vi "TestCloneAPI.vi"() -> ()   [LabVIEW 2018, in "MyPluggableModule.lvlib"]
uses:
  MyPluggableModule.lvlib
  TestInfo.ctl
  <userlib>/NIST/ModuleAdminLib/CloneRegistration/CloneRegistration.lvclass
  <userlib>/NIST/ModuleAdminLib/ModuleAdmin/ModuleAdmin.lvclass/ModuleAdmin.ctl
  <userlib>/NIST/ModuleAdminLib/ModuleAdmin/ModuleAdmin.lvclass
  PluginsShared/clDidInit.ctl
  PluginsShared/clStopArgument.ctl
  <userlib>/NIST/ModuleAdminLib/ModuleAdmin/Accessors/Read CloneRegRef.vi
  <userlib>/NIST/ModuleAdminLib/ModuleAdmin/Accessors/Write CloneRegRef.vi
  PluginsShared/PluginsShared.lvlib
panel:
  in  "btnClear":bool
  in  "btnPref":bool
  in  "Show Panel":bool=TRUE
  in  "Plugin Type":u16(ring) items=["Base Plugin"]
  in  "btnLoadPlugin":bool
  out "File Path Control":path
  in  "btnRequestINIPath":bool
  in  "btnRemove":bool
  out "Status Log":string
  out "Active Modules (Array)":string[](array[string])
  in  "btnAdd":bool
  in  "btnStop":bool
  in  "Select Module":i32(ring)=-1 caption="Select Module to send Request" items=["All"=-1]
  # "Use TestCloneAPI to test the CloneableModule's Application Programming Interface as you develop it.  For each Request and Broadcast event you add to the Clone's Main program, you should add a means of testing it."
  # "Hidden"
  # "Visible"
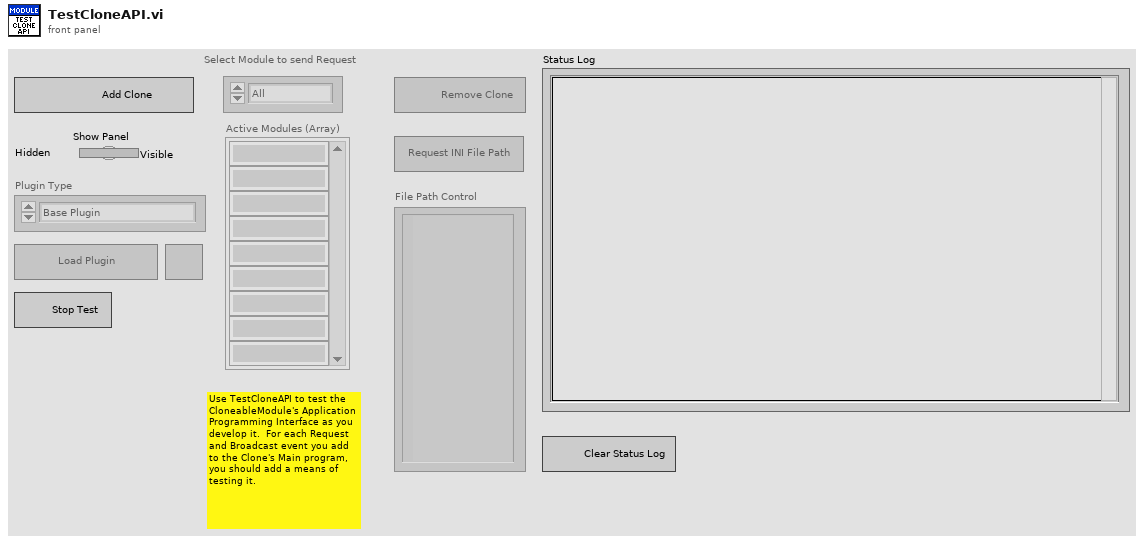
[diagram p1: front panel]
types:
  T1 = typedef "MyPluggableModule.lvlib/TestInfo.ctl" = cluster{"PluginIniFilePaths":path[]}
  T2 = cluster{"Status Log":refnum<vi>, "btnAdd":refnum<vi>, "btnStop":refnum<vi>, "Show Panel":refnum<vi>, "btnClear":refnum<vi>}
  T3 = typedef "PluginsShared.lvlib/clBroadcastEvents.ctl" = cluster{"DidInit":refnum<user-event>, "StatusUpdate":refnum<user-event>, "ErrorReport":refnum<user-event>, "DidStop":refnum<user-event>, "PathToINI":refnum<user-event>, "ReloadINIFiles":refnum<user-event>}
  T4 = enum8{"Enabled", "Disabled", "Disabled and Grayed Out"}
  T5 = typedef "PluginsShared.lvlib/clDidInit.ctl" = cluster{"Init?":bool, "ModuleAdmin":refnum<class "ModuleAdmin.lvclass">}
  T6 = typedef "PluginsShared.lvlib/clStopArgument.ctl" = cluster{"Exit via Stop Module Req?":bool, "Wait for Module to stop?":bool, "ModuleAdmin":refnum<class "ModuleAdmin.lvclass">}
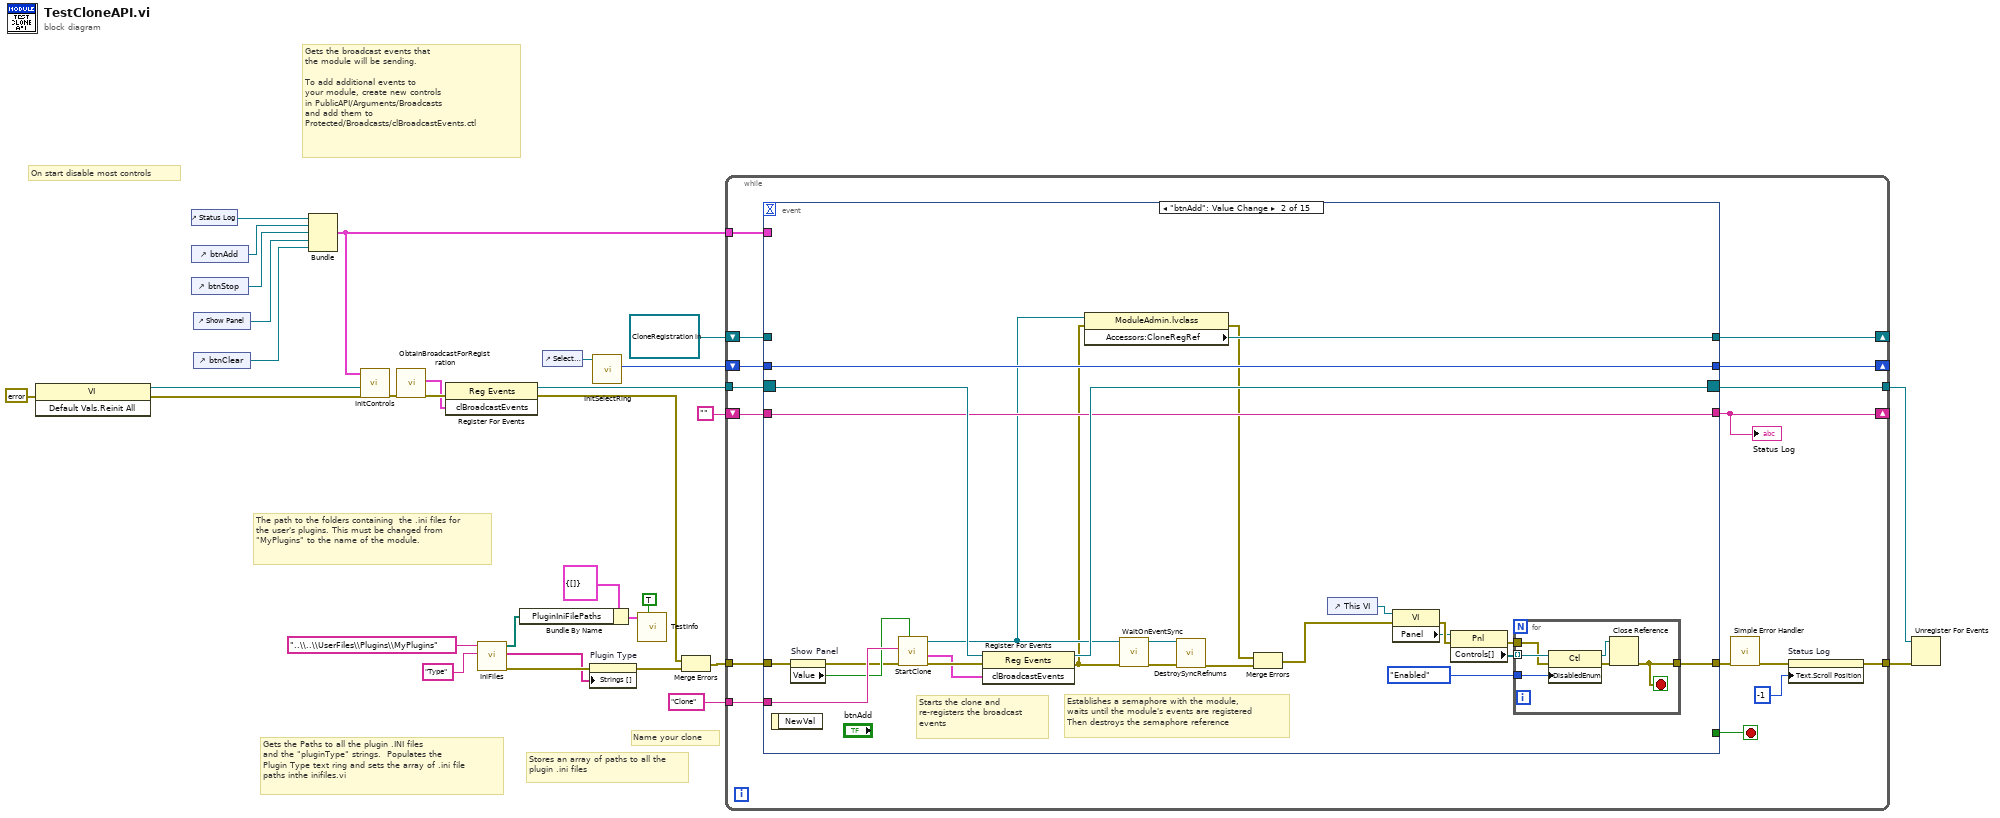
[diagram p0: block diagram]
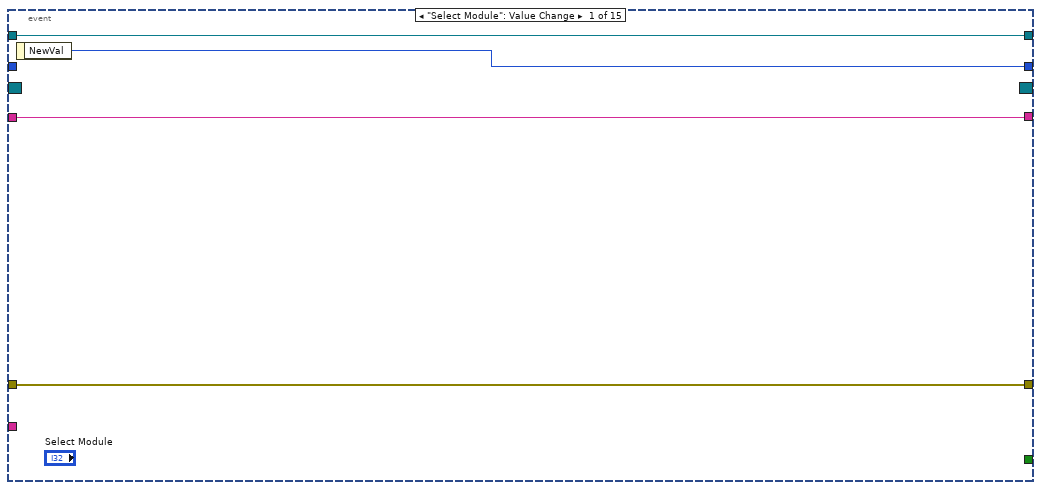
[diagram p2: hidden frame]
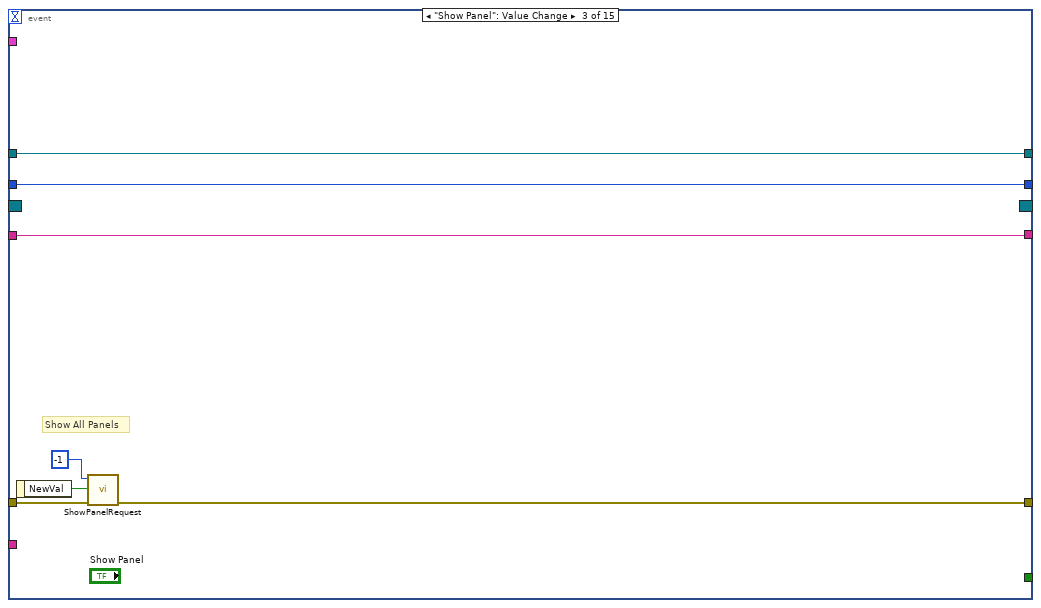
[diagram p3: hidden frame]
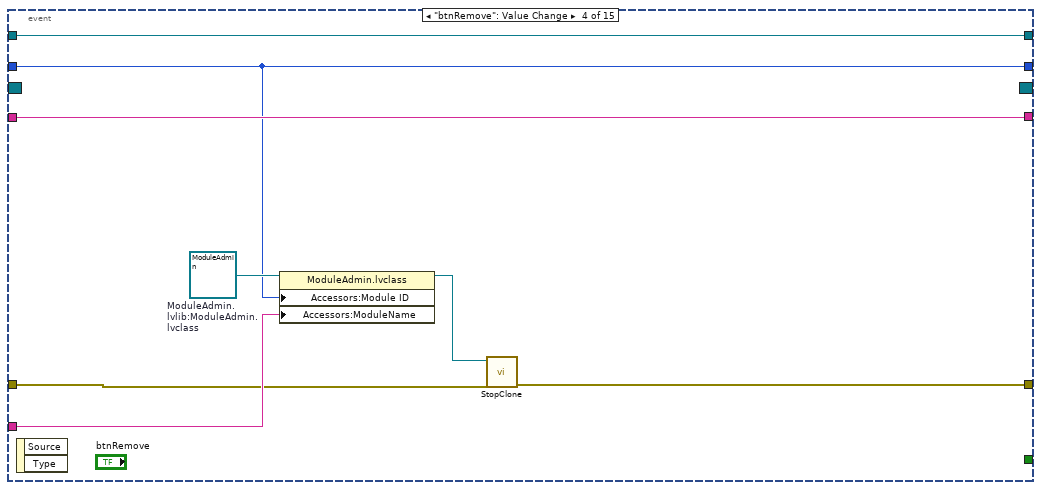
[diagram p4: hidden frame]
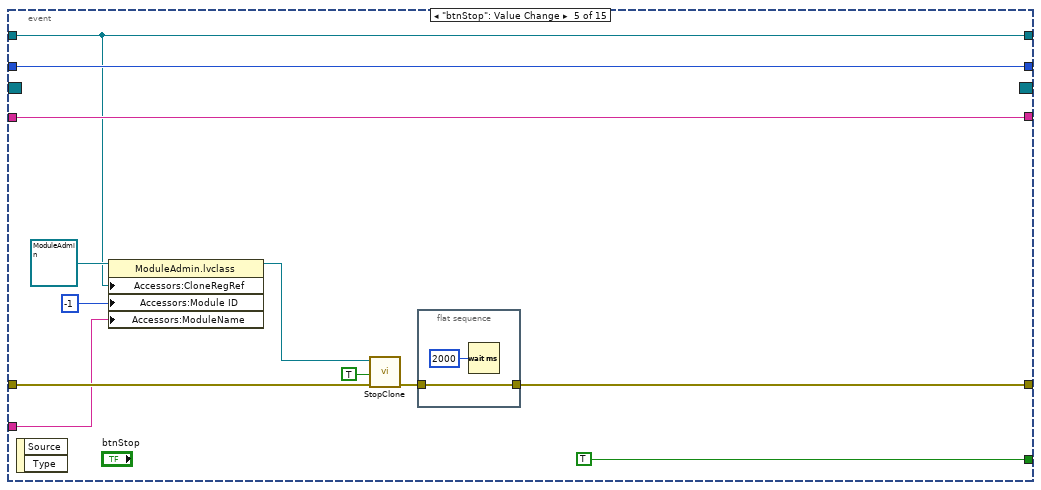
[diagram p5: hidden frame]
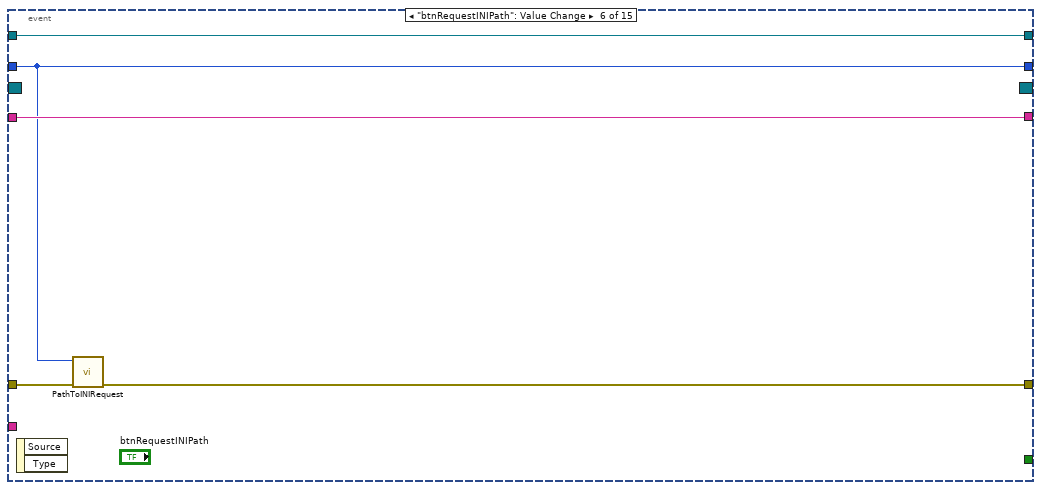
[diagram p6: hidden frame]
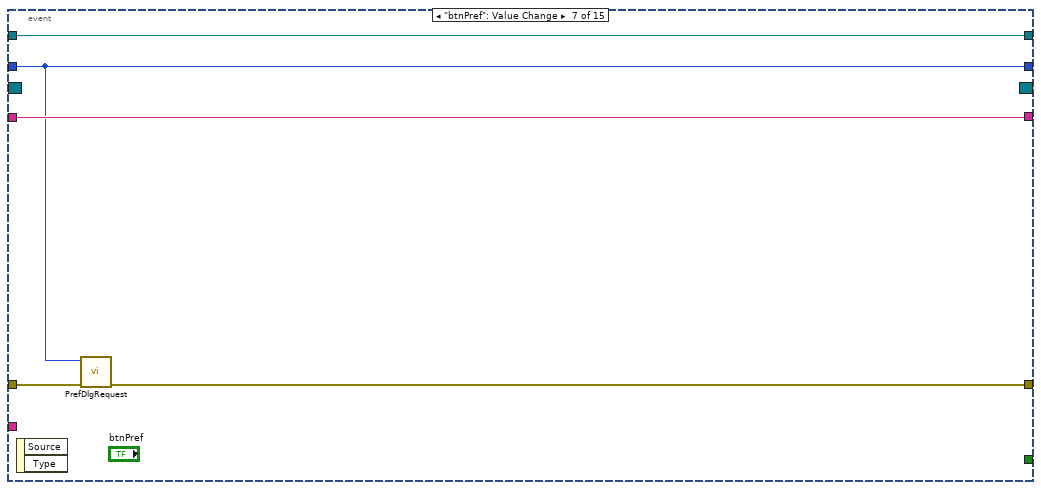
[diagram p7: hidden frame]
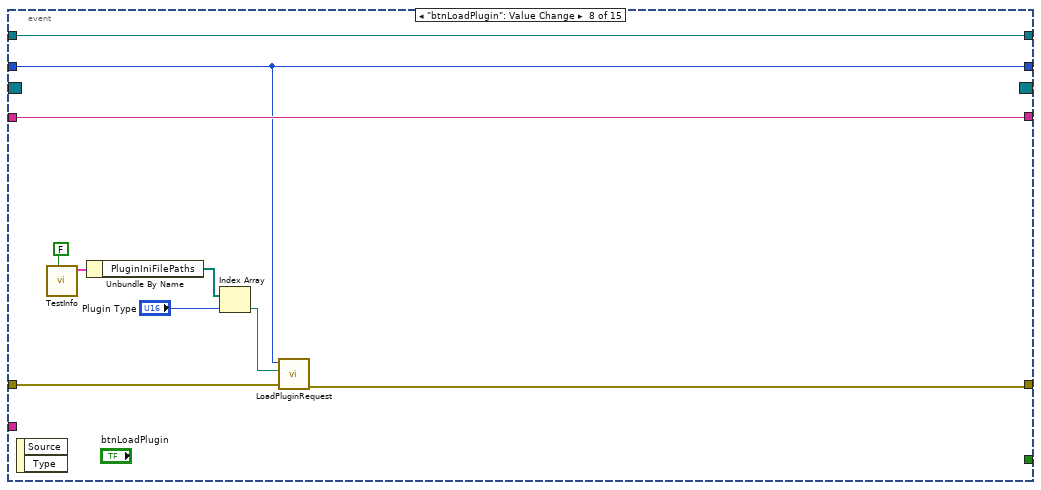
[diagram p8: hidden frame]
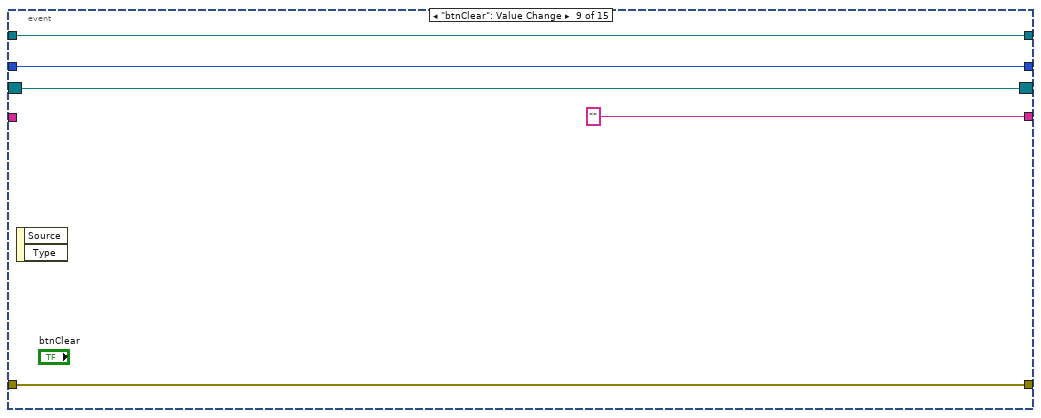
[diagram p9: hidden frame]
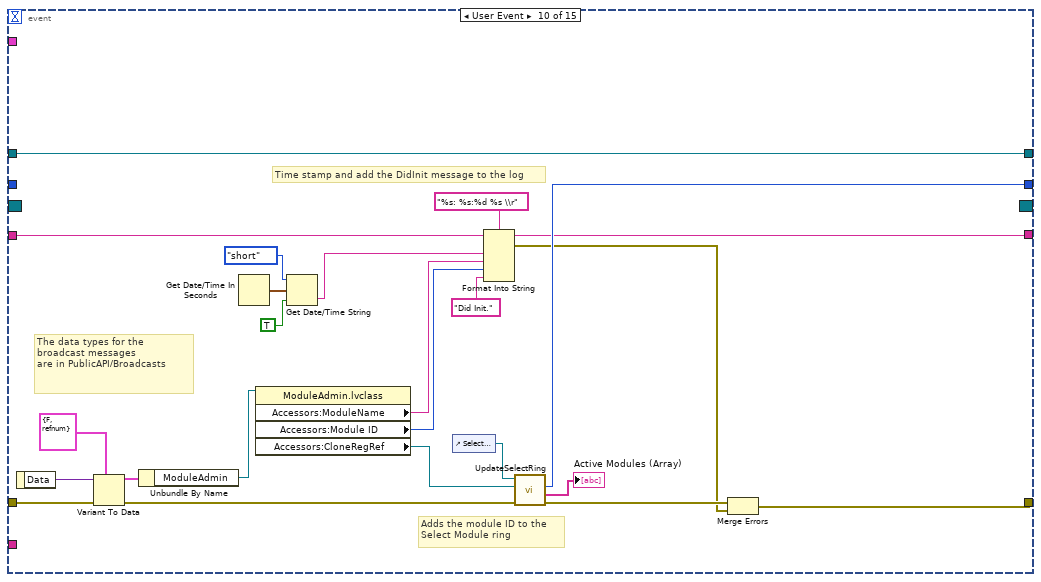
[diagram p10: hidden frame]
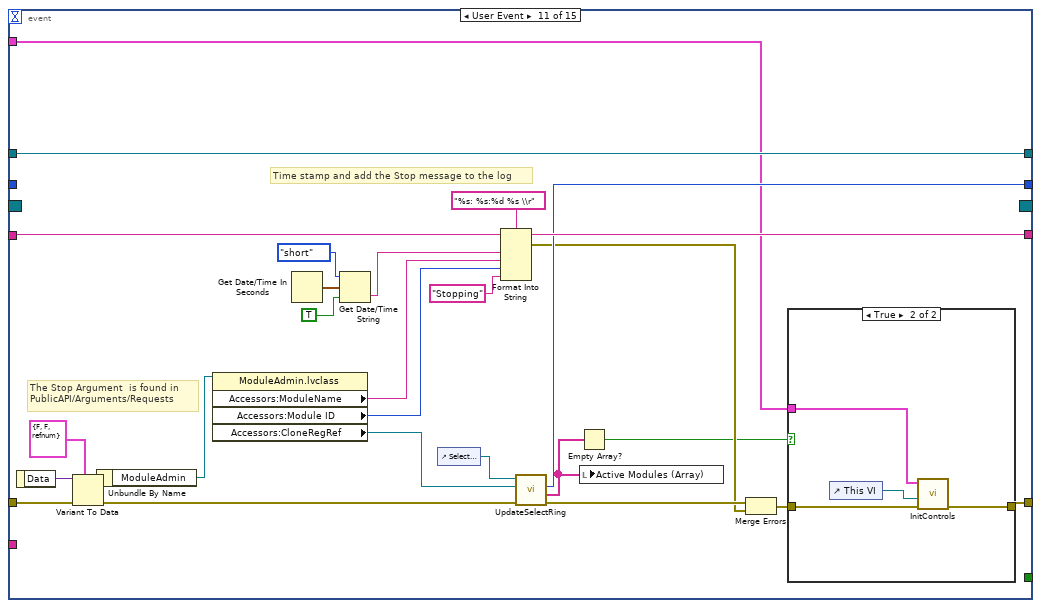
[diagram p11: hidden frame]
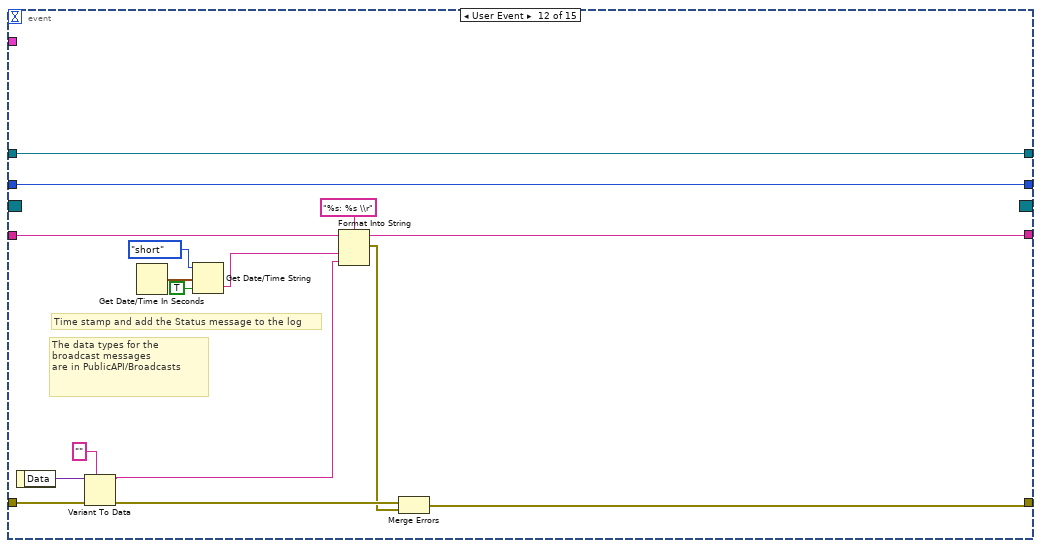
[diagram p13: hidden frame]
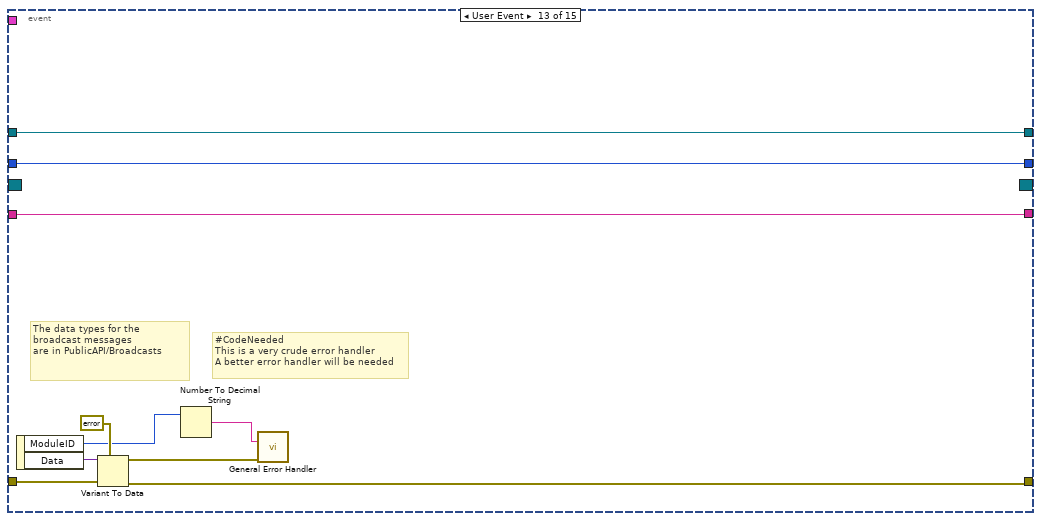
[diagram p14: hidden frame]
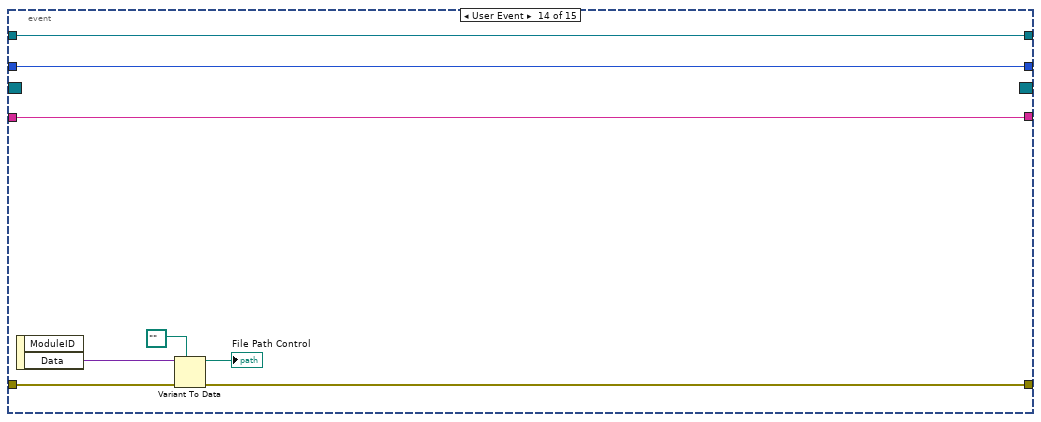
[diagram p15: hidden frame]
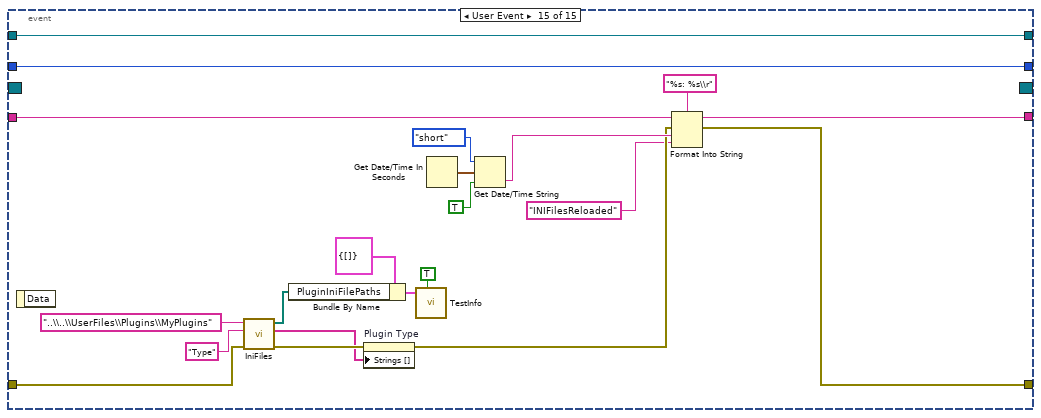
[diagram p16: hidden frame]
diagram:
  # "On start disable most controls"
  # "The path to the folders containing  the .ini files for the user's plugins. This must be changed from \"MyPlugins\" to the name of the module."
  # "Stores an array of paths to all the plugin .ini files"
  # "Gets the Paths to all the plugin .INI files\nand the \"pluginType\" strings.  Populates the \nPlugin Type text ring and sets the array of .ini file\npaths inthe inifiles.vi"
  # "Name your clone"
  # "Gets the broadcast events that\nthe module will be sending.\n\nTo add additional events to\nyour module, create new controls\nin PublicAPI/Arguments/Broadcasts\nand add them to\nProtected/Broadcasts/clBroadcastEvents.ctl"
  n1 = invoke class="VI" method="Default Vals.Reinit All"(error in=errorcluster {"status"=FALSE, "code"=0, "source"=""} ("error in (no error)")) -> (reference out=w10:refnum<vi>, error out=w9:errorcluster)  [unwired: 2 in, 1 out]
  n2 = control-ref of="Status Log"() -> (w6:refnum<vi>)
  n3 = control-ref of="btnAdd"() -> (w5:refnum<vi>)
  n4 = control-ref of="btnStop"() -> (w4:refnum<vi>)
  n5 = control-ref of="Show Panel"() -> (w3:refnum<vi>)
  n6 = control-ref of="btnClear"() -> (w2:refnum<vi>)
  n7 = Bundle("Status Log"=w6, "btnAdd"=w5, "btnStop"=w4, "Show Panel"=w3, "btnClear"=w2) -> (w1:T2)  [unwired: 1 in]
  n8 = call "InitControls.vi"("error in (no error)"=w9, "TestCloneAPI Reference"=w10, "Cluster Of Controls to Enable"=w1) -> ("error out"=w8:errorcluster)  [unwired: 8 in]
  n9 = call "ObtainBroadcastForRegistration.vi"("error in (no error)"=w8) -> ("error out"=w29:errorcluster, "clBroadcastEvents"=w28:T3)  [unwired: 9 in]
  n10 = register-events(error in=w29, w28) -> (reference out=w26:refnum<event-registration>, error out=w27:errorcluster)  [unwired: 1 in]
  n11 = call "IniFiles.vi"("iniKey"="Type", "name or relative path"="..\\..\\UserFiles\\Plugins\\MyPlugins") -> ("error out"=w23:errorcluster, "Types"=w22:string[], "IniFilePaths"=w21:path[])  [unwired: 7 in]
  n12 = Bundle By Name(cluster=T1 {"PluginIniFilePaths"=[]} ("TestInfo"), "PluginIniFilePaths"=w21) -> (w20:T1)
  n13 = control-ref of="Select Module"() -> (w31:refnum<vi>)
  n14 = property on="Plugin Type" class="Ring (strict)"(error in=w23, "Strings []"=w22) -> (error out=w17:errorcluster)  [unwired: 1 in, 1 out]
  n15 = call "InitSelectRing.vi"("Ring Refnum"=w31) -> ("Module Ring Value"=w30:i32)  [unwired: 9 in, 1 out]
  n16 = call "TestInfo.vi"("Set (f)"=TRUE, "TestInfo 2"=w20) -> ()  [unwired: 9 in, 1 out]
  n17 = Merge Errors(w27, w17) -> (w18:errorcluster)
  n18 = while {
    shift-right: [w46] -> _
    shift-left: w30 -> [w47]
    tunnel: w18 -> [w44]
    tunnel: w26 -> [w42]
    tunnel: [w33] -> w13
    shift-right: [w41] -> _
    shift-left: "" -> [w40]
    tunnel: "Clone" ("ModuleName") -> [w39]
    tunnel: [w38] -> w12
    shift-right: [w37] -> _
    shift-left: refnum<data-value> refnum ("Accessors:CloneRegRef") -> [w36]
    tunnel: w1 -> [w32]
    stop <- w45 stop-if-true
    n19 = event shown="[1] \"btnAdd\": Value Change" {
      selector: w42 -> [_ w70 _ _ _ _ _ _ w134 _ _ _ _ _ _]
      dyn-events: [_ w69 _ _ _ _ _ _ w134 _ _ _ _ _ _] -> w38
      timeout: _ -> [_ _ _ _ _ _ _ _ _ _ _ _ _ _ _]
      tunnel: w47 -> [_ w76 w85 w92 w109 w115 w120 w128 w133 _ _ w208 w212 w225 w246]
      tunnel: [w51 w76 w85 w92 w109 w115 w120 w128 w133 w155 w175 w208 w212 w225 w246] -> w46
      tunnel: [_ _ _ _ TRUE _ _ _ _ _ _ _ _ _ _] -> w45
      tunnel: w44 -> [w49 w53 w88 w90 w107 w114 w119 w130 w136 w160 w183 w205 w217 w221 w237]
      tunnel: [w49 w60 w86 w91 w98 w113 w118 w129 w136 w144 w163 w198 w216 w220 w229] -> w43
      tunnel: [w50 w68 w84 w97 w105 w116 w121 w131 "" w148 w180 w201 w211 w226 w228] -> w41
      tunnel: w40 -> [w50 w68 w84 w97 w105 w116 w121 w131 _ w147 w181 w207 w211 w226 w231]
      tunnel: w39 -> [_ w67 _ w95 w103 _ _ _ _ _ _ _ _ _ _]
      tunnel: [w48 w64 w83 w93 w100 w112 w117 w122 w132 w137 w166 w193 w209 w219 w247] -> w37
      tunnel: w36 -> [w48 _ w83 w93 w100 w112 w117 w122 w132 w137 w166 w193 w209 w219 w247]
      tunnel: w32 -> [_ _ _ _ _ _ _ _ _ _ w161 _ _ _ _]
      event "Select Module": Value Change {
        n20 = event-data() -> ("NewVal"=w51:i32)  [unwired: 1 in]
      }
      event "btnAdd": Value Change {
        # "Establishes a semaphore with the module,\nwaits until the module's events are registered\nThen destroys the semaphore reference"
        # "Starts the clone and\nre-registers the broadcast \nevents"
        n21 = event-data() -> ()  [unwired: 1 in, 1 out]
        n22 = property on="Show Panel" class="Bool (strict)"(error in=w53) -> (error out=w52:errorcluster, "Value"=w66:bool)  [unwired: 1 in, 1 out]
        n23 = call "StartClone.vi"("ShowPanel? (f)"=w66, "error in (no error)"=w52, "ModuleName"=w67) -> ("error out"=w75:errorcluster, "clBroadcastEvents"=w72:T3, "ModuleAdmin"=w65:refnum<class "ModuleAdmin.lvclass">)  [unwired: 6 in]
        n24 = register-events(reference=w70, error in=w75, w72) -> (reference out=w69:refnum<event-registration>, error out=w63:errorcluster)
        n25 = property class="ModuleAdmin.lvclass"(reference=w65, error in=w63) -> (error out=w62:errorcluster, "Accessors:CloneRegRef"=w64:refnum<data-value>)  [unwired: 1 out]
        n26 = call <userlib>:"WaitOnEventSync.vi"("error in (no error)"=w63, "ModuleAdmin"=w65) -> ("error out"=w74:errorcluster, "ModuleAdmin"=w73:refnum<class "ModuleAdmin.lvclass">)  [unwired: 8 in]
        n27 = call <userlib>:"DestroySyncRefnums.vi"("error in (no error)"=w74, "ModuleAdmin"=w73) -> ("error out"=w71:errorcluster)  [unwired: 9 in]
        n28 = Merge Errors(w62, w71) -> (w61:errorcluster)
        n29 = control-ref of="This VI"() -> (w54:refnum<vi>)
        n30 = property class="VI"(reference=w54, error in=w61) -> (error out=w57:errorcluster, "Panel"=w55:refnum<vi>)  [unwired: 1 out]
        n31 = property class="Pnl"(reference=w55, error in=w57) -> (error out=w58:errorcluster, "Controls[]"=w56:refnum<vi>[])  [unwired: 1 out]
        n32 = for {
          tunnel: w56 -> [w82] mode=indexing
          tunnel: w58 -> [w81]
          tunnel: [w78] -> w60
          tunnel: T4."Enabled" ("Disabled") -> [w77]
          stop <- w78 stop-if-true
          n33 = property class="Ctl"(reference=w82, error in=w81, "DisabledEnum"=w77) -> (reference out=w79:refnum<vi>, error out=w80:errorcluster)
          n34 = Close Reference(reference=w79, error in (no error)=w80) -> (error out=w78:errorcluster)
        }
      }
      event "Show Panel": Value Change {
        # "Show All Panels"
        n35 = event-data() -> ("NewVal"=w89:bool)  [unwired: 1 in]
        n36 = call "ShowPanelRequest.vi"("error in (no error)"=w88, "ShowPanel?"=w89, "ModuleID"=-1) -> ("error out"=w86:errorcluster)  [unwired: 8 in]
      }
      event "btnRemove": Value Change {
        w96 = refnum<class "ModuleAdmin.lvclass"> refnum  # ModuleAdmin.lvlib:ModuleAdmin.lvclass
        n37 = event-data() -> ()  [unwired: 1 in, 2 out]
        n38 = property class="ModuleAdmin.lvclass"(reference=w96, "Accessors:Module ID"=w92, "Accessors:ModuleName"=w95) -> (reference out=w94:refnum<class "ModuleAdmin.lvclass">)  [unwired: 1 in, 1 out]
        n39 = call "StopClone.vi"("error in (no error)"=w90, "ModuleAdmin"=w94) -> ("error out"=w91:errorcluster)  [unwired: 9 in]
      }
      event "btnStop": Value Change {
        n40 = event-data() -> ()  [unwired: 1 in, 2 out]
        n41 = property class="ModuleAdmin.lvclass"(reference=refnum<class "ModuleAdmin.lvclass"> refnum ("ModuleAdmin.lvlib:ModuleAdmin.lvclass"), "Accessors:CloneRegRef"=w100, "Accessors:Module ID"=-1 ("Module ID"), "Accessors:ModuleName"=w103) -> (reference out=w102:refnum<class "ModuleAdmin.lvclass">)  [unwired: 1 in, 1 out]
        n42 = call "StopClone.vi"("error in (no error)"=w107, "Wait for Module to stop?"=TRUE, "ModuleAdmin"=w102) -> ("error out"=w99:errorcluster)  [unwired: 8 in]
        n43 = flat-sequence {
          tunnel: w99 -> [w110]
          tunnel: [w110] -> w98
          frame #0 {
            n44 = Wait (ms)(milliseconds to wait=u32 2000) -> ()  [unwired: 1 out]
          }
        }
      }
      event "btnRequestINIPath": Value Change {
        n45 = event-data() -> ()  [unwired: 1 in, 2 out]
        n46 = call "PathToINIRequest.vi"("error in (no error)"=w114, "ModuleID"=w115) -> ("error out"=w113:errorcluster)  [unwired: 9 in]
      }
      event "btnPref": Value Change {
        n47 = event-data() -> ()  [unwired: 1 in, 2 out]
        n48 = call "PrefDlgRequest.vi"("error in (no error)"=w119, "ModuleID"=w120) -> ("error out"=w118:errorcluster)  [unwired: 9 in]
      }
      event "btnLoadPlugin": Value Change {
        n49 = event-data() -> ()  [unwired: 1 in, 2 out]
        n50 = call "TestInfo.vi"("Set (f)"=FALSE) -> ("TestInfo"=w126:T1)  [unwired: 10 in]
        n51 = Unbundle By Name(w126) -> ("PluginIniFilePaths"=w125:path[])
        n52 = Index Array(array=w125, index="Plugin Type") -> (element=w123:path)
        n53 = call "LoadPluginRequest.vi"("error in (no error)"=w130, "PathToPluginINI"=w123, "ModuleID"=w128) -> ("error out"=w129:errorcluster)  [unwired: 8 in]
      }
      event "btnClear": Value Change {
        n54 = event-data() -> ()  [unwired: 1 in, 2 out]
      }
      event User Event {
        # "Adds the module ID to the \nSelect Module ring"
        # "Time stamp and add the DidInit message to the log"
        # "The data types for the broadcast messages\nare in PublicAPI/Broadcasts"
        n55 = event-data() -> ("Data"=w159:variant)  [unwired: 1 in]
        n56 = Variant To Data(error in=w160, type=T5 {"Init?"=FALSE, "ModuleAdmin"=refnum} ("clDidInit"), Variant=w159) -> (data=w152:T5, error out=w157:errorcluster)
        n57 = Unbundle By Name(w152) -> ("ModuleAdmin"=w142:refnum<class "ModuleAdmin.lvclass">)
        n58 = Get Date/Time In Seconds() -> (seconds since 1Jan1904=w150:timestamp)
        n59 = property class="ModuleAdmin.lvclass"(reference=w142) -> ("Accessors:ModuleName"=w140:string, "Accessors:Module ID"=w139:i32, "Accessors:CloneRegRef"=w138:refnum<data-value>)  [unwired: 1 in, 2 out]
        n60 = Get Date/Time String(date format (0)=enum16{"short", "long", "abbreviated"}."short", seconds (now)=w150, want seconds? (F)=TRUE) -> (time string=w153:string)  [unwired: 1 out]
        n61 = control-ref of="Select Module"() -> (w156:refnum<vi>)
        n62 = Format Into String(format string="%s: %s:%d %s \\r", initial string=w147, w153, w140, w139, "Did Init.") -> (resulting string=w148:string, error out=w145:errorcluster)  [unwired: 1 in]
        n63 = call "UpdateSelectRing.vi"("error in (no error)"=w157, "CloneRegRef"=w138, "Ring Refnum"=w156) -> ("error out"=w146:errorcluster, "ActiveModules"=→"Active Modules (Array)":string[], "Module Ring Value"=w155:i32)  [unwired: 6 in]
        n64 = Merge Errors(w146, w145) -> (w144:errorcluster)
      }
      event User Event {
        # "Time stamp and add the Stop message to the log"
        # "The Stop Argument  is found in\nPublicAPI/Arguments/Requests"
        n65 = event-data() -> ("Data"=w182:variant)  [unwired: 1 in]
        n66 = Variant To Data(error in=w183, type=T6 {"Exit via Stop Module Req?"=FALSE, "Wait for Module to stop?"=FALSE, "ModuleAdmin"=refnum} ("Stop Argument"), Variant=w182) -> (data=w178:T6, error out=w177:errorcluster)
        n67 = Unbundle By Name(w178) -> ("ModuleAdmin"=w171:refnum<class "ModuleAdmin.lvclass">)
        n68 = property class="ModuleAdmin.lvclass"(reference=w171) -> ("Accessors:ModuleName"=w169:string, "Accessors:Module ID"=w168:i32, "Accessors:CloneRegRef"=w167:refnum<data-value>)  [unwired: 1 in, 2 out]
        n69 = Get Date/Time In Seconds() -> (seconds since 1Jan1904=w185:timestamp)
        n70 = Get Date/Time String(date format (0)=enum16{"short", "long", "abbreviated"}."short", seconds (now)=w185, want seconds? (F)=TRUE) -> (time string=w187:string)  [unwired: 1 out]
        n71 = control-ref of="Select Module"() -> (w176:refnum<vi>)
        n72 = Format Into String(format string="%s: %s:%d %s \\r", initial string=w181, w187, w169, w168, "Stopping") -> (resulting string=w180:string, error out=w173:errorcluster)  [unwired: 1 in]
        n73 = call "UpdateSelectRing.vi"("error in (no error)"=w177, "CloneRegRef"=w167, "Ring Refnum"=w176) -> ("error out"=w174:errorcluster, "ActiveModules"=w165:string[], "Module Ring Value"=w175:i32)  [unwired: 6 in]
        n74 = Empty Array?(array=w165) -> (empty?=w162:bool)
        n75 = local write "Active Modules (Array)"(w165) -> ()
        n76 = Merge Errors(w174, w173) -> (w164:errorcluster)
        n77 = case shown="True" w162 {
          tunnel: w164 -> [w188 w192]
          tunnel: [w188 w191] -> w163
          tunnel: w161 -> [_ w189]
          frame False {
          }
          frame True {
            n78 = control-ref of="This VI"() -> (w190:refnum<vi>)
            n79 = call "InitControls.vi"("error in (no error)"=w192, "TestCloneAPI Reference"=w190, "Cluster Of Controls to Enable"=w189) -> ("error out"=w191:errorcluster)  [unwired: 8 in]
          }
        }
      }
      event User Event {
        # "Time stamp and add the Status message to the log"
        # "The data types for the broadcast messages\nare in PublicAPI/Broadcasts"
        n80 = event-data() -> ("Data"=w204:variant)  [unwired: 1 in]
        n81 = Variant To Data(error in=w205, type="" ("clStatUpdate"), Variant=w204) -> (data=w194:string, error out=w200:errorcluster)
        n82 = Get Date/Time In Seconds() -> (seconds since 1Jan1904=w202:timestamp)
        n83 = Get Date/Time String(date format (0)=enum16{"short", "long", "abbreviated"}."short", seconds (now)=w202, want seconds? (F)=TRUE) -> (time string=w195:string)  [unwired: 1 out]
        n84 = Format Into String(format string="%s: %s \\r", initial string=w207, w195, w194) -> (resulting string=w201:string, error out=w199:errorcluster)  [unwired: 1 in]
        n85 = Merge Errors(w200, w199) -> (w198:errorcluster)
      }
      event User Event {
        # "#CodeNeeded\nThis is a very crude error handler\nA better error handler will be needed"
        # "The data types for the broadcast messages\nare in PublicAPI/Broadcasts"
        n86 = event-data() -> ("ModuleID"=w214:i32, "Data"=w218:variant)  [unwired: 1 in]
        n87 = Variant To Data(error in=w217, type=errorcluster {"status"=FALSE, "code"=0, "source"=""} ("Cluster"), Variant=w218) -> (data=w210:errorcluster, error out=w216:errorcluster)
        n88 = Number To Decimal String(number=w214) -> (decimal integer string=w213:string)  [unwired: 1 in]
        n89 = call <vilib>:"General Error Handler.vi"("[error source] (\" \")"=w213, "error in (no error)"=w210) -> ()  [unwired: 9 in, 5 out]
      }
      event User Event {
        n90 = event-data() -> ("Data"=w223:variant)  [unwired: 1 in, 1 out]
        n91 = Variant To Data(error in=w221, type=path "" ("Path"), Variant=w223) -> (data=→"File Path Control":path, error out=w220:errorcluster)
      }
      event User Event {
        n92 = event-data() -> ()  [unwired: 1 in, 1 out]
        n93 = call "IniFiles.vi"("error in"=w237, "iniKey"="Type", "name or relative path"="..\\..\\UserFiles\\Plugins\\MyPlugins") -> ("error out"=w245:errorcluster, "Types"=w244:string[], "IniFilePaths"=w243:path[])  [unwired: 6 in]
        n94 = Bundle By Name(cluster=T1 {"PluginIniFilePaths"=[]} ("TestInfo"), "PluginIniFilePaths"=w243) -> (w242:T1)
        n95 = property on="Plugin Type" class="Ring (strict)"(error in=w245, "Strings []"=w244) -> (error out=w230:errorcluster)  [unwired: 1 in, 1 out]
        n96 = call "TestInfo.vi"("Set (f)"=TRUE, "TestInfo 2"=w242) -> ()  [unwired: 9 in, 1 out]
        n97 = Get Date/Time In Seconds() -> (seconds since 1Jan1904=w234:timestamp)
        n98 = Get Date/Time String(date format (0)=enum16{"short", "long", "abbreviated"}."short", seconds (now)=w234, want seconds? (F)=TRUE) -> (time string=w236:string)  [unwired: 1 out]
        n99 = Format Into String(format string="%s: %s\\r", initial string=w231, error in=w230, w236, "INIFilesReloaded") -> (resulting string=w228:string, error out=w229:errorcluster)
      }
    }
    "Status Log" <- w41
    n100 = call <vilib>:"Simple Error Handler.vi"("error in (no error)"=w43) -> ("error out"=w34:errorcluster)  [unwired: 4 in, 4 out]
    n101 = property on="Status Log" class="Str"(error in=w34, "Text.Scroll Position"=-1) -> (error out=w33:errorcluster)  [unwired: 1 in, 1 out]
  }
  n102 = Unregister For Events(event registration refnum=w12, error in=w13) -> ()  [unwired: 1 out]
